vi "Acceleration Sensor-DM.vi"(2 "NXT":T3={"error"={"status"=FALSE, "code"=0, "source"=""}, "address"="", "NXT #"=-1, "Show Error"=TRUE, "Connection"=4} {"Connection" items=["USB", "Bluetooth", "USB then Bluetooth", "Last Connection", "Preference"]}, 3 "Input Port":T2 items=["Port 1", "Port 2", "Port 3", "Port 4"]) -> (1 "Output of Acceleration Sensor":T1, 4 "NXT dup":T3={"error"={"status"=FALSE, "code"=0, "source"=""}, "address"="", "NXT #"=-1, "Show Error"=TRUE, "Connection"=4} caption="NXT" {"Connection" items=["USB", "Bluetooth", "USB then Bluetooth", "Last Connection", "Preference"]})   [LabVIEW 2009]
uses:
  <vilib>/NXT/Subs/LVHSConnector.ctl
  <vilib>/NXT/Block Support/NXT_InputPort.ctl
  <vilib>/NXT/Block Support/HWPage.SensorType.ctl
  <vilib>/NXT/Block Support/HWPage.SensorMode.ctl
panel:
  out "Status":bool caption="Success?"
  out "Z Accel":i16
  out "Y Accel":i16
  out "X Accel":i16
  out "Z Tilt":i16
  out "Y Tilt":i16
  out "X Tilt":i16
  # "mindsensors.com\nCopyright (c) 2009 by mindsensors.com\nEmail: info (<at>) mindsensors (<dot>) com\n\nThis program is free software. You can redistribute it and/or modify\nit under the terms of the GNU General Public License as published by\nthe Free Software Foundation; version 3 of the License.\nRead the license at: http://www.gnu.org/licenses/gpl.txt"
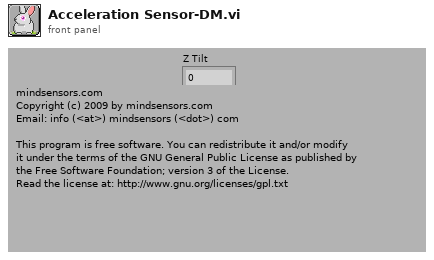
[diagram p1: front panel]
types:
  T1 = cluster{"X Tilt":i16, "Y Tilt":i16, "Z Tilt":i16, "X Accel":i16, "Y Accel":i16, "Z Accel":i16, "Status (boolean)":bool}
  T2 = typedef "NXT_InputPort.ctl" = u8
  T3 = typedef "LVHSConnector.ctl" = cluster{"error":errorcluster, "address":string, "NXT #":i32, "Show Error":bool, "Connection":u16}
  T4 = typedef "HWPage.SensorType.ctl" = u8
  T5 = typedef "HWPage.SensorMode.ctl" = u8
  T6 = cluster{i16, i16, i16, i16, i16, i16, "Status":bool}
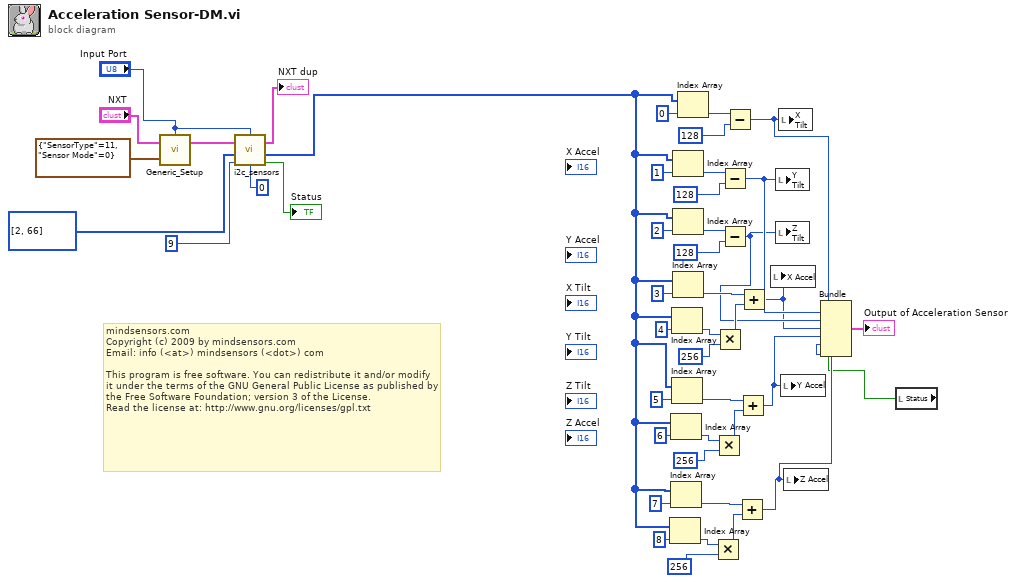
[diagram p0: block diagram]
diagram:
  # "mindsensors.com\nCopyright (c) 2009 by mindsensors.com\nEmail: info (<at>) mindsensors (<dot>) com\n\nThis program is free software. You can redistribute it and/or modify\nit under the terms of the GNU General Public License as published by\nthe Free Software Foundation; version 3 of the License.\nRead the license at: http://www.gnu.org/licenses/gpl.txt"
  n1 = call <vilib>:"Generic_Setup.vi"("Sensor Setup"=cluster{"SensorType":T4, "Sensor Mode":T5} {"SensorType"=11, "Sensor Mode"=0}, "NXT"="NXT", "Port"="Input Port") -> ("NXT"=w40:T3)  [unwired: 1 out]
  n2 = call <vilib>:"i2c_sensors.vi"("Return Length"=u8 9, "Bytes to Write"=u8[] [2, 66] ("Parameters"), "Wait (msec)"=u32 0, "NXT"=w40, "Port"="Input Port") -> ("Success?"=→"Status":bool, "Bytes read"=w39:u8[], "NXT"=→"NXT dup":T3)
  n3 = Index Array(array=w39, index=8) -> (element=w14:u8)
  n4 = Index Array(array=w39, index=6) -> (element=w19:u8)
  n5 = Index Array(array=w39, index=7) -> (element=w16:u8)
  n6 = Index Array(array=w39, index=4) -> (element=w33:u8)
  n7 = Index Array(array=w39, index=5) -> (element=w21:u8)
  n8 = Index Array(array=w39, index=1) -> (element=w27:u8)
  n9 = Index Array(array=w39, index=2) -> (element=w24:u8)
  n10 = Index Array(array=w39, index=3) -> (element=w35:u8)
  n11 = Index Array(array=w39, index=0) -> (element=w31:u8)
  n12 = Multiply(x=w14, y=i16 256) -> (x*y=w15:i16)
  n13 = Multiply(x=w19, y=i16 256) -> (x*y=w20:i16)
  n14 = Multiply(x=w33, y=i16 256) -> (x*y=w34:i16)
  n15 = Subtract(x=w27, y=i16 128) -> (x-y=w9:i16)
  n16 = Subtract(x=w24, y=i16 128) -> (x-y=w8:i16)
  n17 = Subtract(x=w31, y=i16 128) -> (x-y=w10:i16)
  n18 = Add(x=w16, y=w15) -> (x+y=w5:i16)
  n19 = Add(x=w21, y=w20) -> (x+y=w6:i16)
  n20 = Add(x=w35, y=w34) -> (x+y=w7:i16)
  n21 = local write "X Accel"(w7) -> ()
  n22 = local write "Y Tilt"(w9) -> ()
  n23 = local write "Z Tilt"(w8) -> ()
  n24 = local write "X Tilt"(w10) -> ()
  n25 = local write "Y Accel"(w6) -> ()
  n26 = local write "Z Accel"(w5) -> ()
  n27 = local read "Status"() -> (w2:bool)
  n28 = Bundle(w10, w9, w8, w7, w6, w5, "Status"=w2) -> (→"Output of Acceleration Sensor":T6)  [unwired: 1 out]
